vi "Prog6.vi"() -> ()   [LabVIEW 2021]
panel:
  out "size(s)":i32
  out "Array 2":string[](array[string])
  out "Array":string[](array[string])
  out "string 2":string
  out "string":string
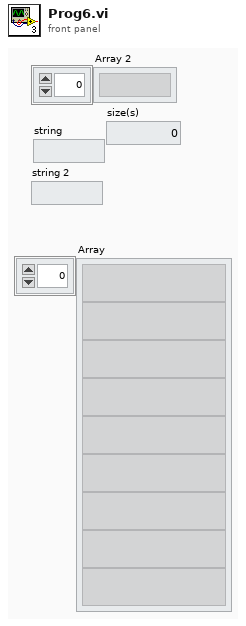
[diagram p1: front panel]
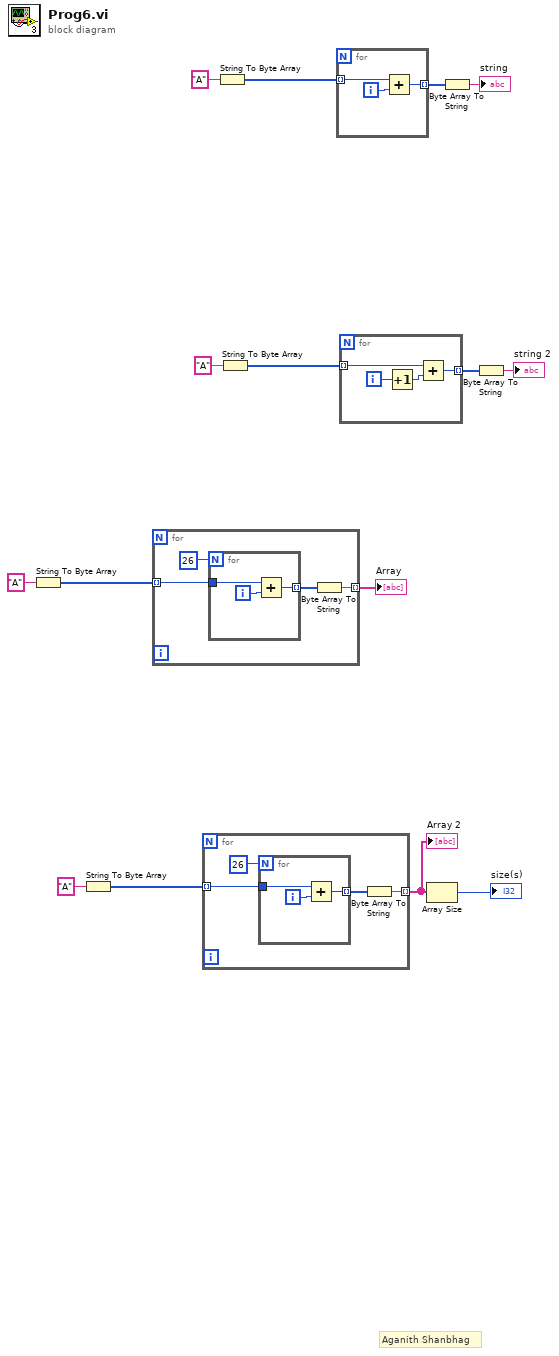
[diagram p0: block diagram]
diagram:
  # "Aganith Shanbhag"
  n1 = String To Byte Array(string="A") -> (unsigned byte array=w5:u8[])
  n2 = String To Byte Array(string="A") -> (unsigned byte array=w3:u8[])
  n3 = for {
    tunnel: [w18] -> w7 mode=indexing
    tunnel: w5 -> [w16] mode=indexing
    n4 = for {
      N: 26 -> [_]
      tunnel: w16 -> [w22]
      tunnel: [w21] -> w19 mode=indexing
      i -> [w20]
      n5 = Add(x=w22, y=w20) -> (x+y=w21:i32)
    }
    n6 = Byte Array To String(unsigned byte array=w19) -> (string=w18:string)
  }
  "Array" <- w7
  n7 = for {
    tunnel: [w25] -> w2 mode=indexing
    tunnel: w3 -> [w23] mode=indexing
    n8 = for {
      N: 26 -> [_]
      tunnel: w23 -> [w29]
      tunnel: [w28] -> w26 mode=indexing
      i -> [w27]
      n9 = Add(x=w29, y=w27) -> (x+y=w28:i32)
    }
    n10 = Byte Array To String(unsigned byte array=w26) -> (string=w25:string)
  }
  "Array 2" <- w2
  n11 = String To Byte Array(string="A") -> (unsigned byte array=w12:u8[])
  n12 = String To Byte Array(string="A") -> (unsigned byte array=w8:u8[])
  n13 = for {
    tunnel: w12 -> [w32] mode=indexing
    tunnel: [w31] -> w14 mode=indexing
    i -> [w30]
    n14 = Add(x=w32, y=w30) -> (x+y=w31:i32)
  }
  n15 = for {
    tunnel: w8 -> [w36] mode=indexing
    tunnel: [w35] -> w10 mode=indexing
    i -> [w33]
    n16 = Increment(x=w33) -> (x+1=w34:i32)
    n17 = Add(x=w36, y=w34) -> (x+y=w35:i32)
  }
  n18 = Array Size(array=w2) -> (size(s)=→"size(s)":i32)
  n19 = Byte Array To String(unsigned byte array=w14) -> (string=→"string":string)
  n20 = Byte Array To String(unsigned byte array=w10) -> (string=→"string 2":string)
